vi "Launch Data Validation Example.vi"(4 "Error In":errorcluster, 7 "Data Passback Event":refnum<user-event>) -> (0 "Error Out":errorcluster)   [LabVIEW 2014, in "Dialog Boxes.lvlib"]
uses:
  Dialog Boxes.lvlib
  _dialogs/Data Validation Example.vi
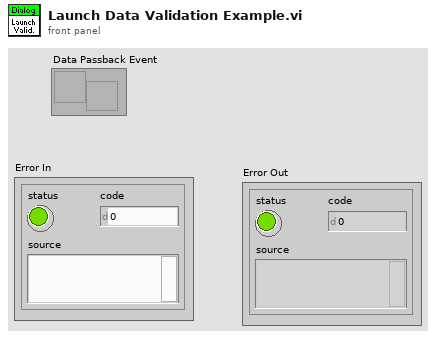
[diagram p1: front panel]
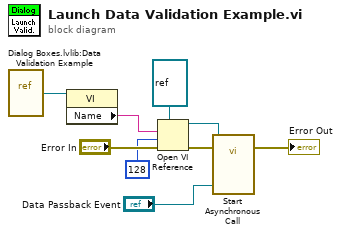
[diagram p0: block diagram]
diagram:
  n1 = vi-ref "Dialog Boxes.lvlib:Data Validation Example.vi"() -> (w9:refnum<vi>)
  n2 = property class="VI"(reference=w9) -> ("Name"=w8:string)  [unwired: 1 in, 2 out]
  n3 = Open VI Reference(type specifier VI Refnum (for type only)=refnum<vi> refnum, vi path=w8, options=128, error in (no error)="Error In") -> (vi reference=w5:refnum<vi>, error out=w6:errorcluster)  [unwired: 2 in]
  n4 = call-by-ref "Start Asynchronous Call"(reference=w5, error in=w6, "Passback Data"="Data Passback Event") -> (error out=→"Error Out":errorcluster)  [unwired: 11 in, 1 out]
